vi "ni_home.vi"(8 "error in":errorcluster) -> (0 "error out":errorcluster)   [LabVIEW 2014]
uses:
  <vilib>/Motion/FlexMotion/CustomControls/CustomControls.llb/Axis # (8 axes).flx
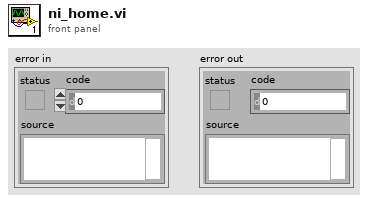
[diagram p1: front panel]
types:
  T1 = typedef "Board Id" = u8
  T2 = enum16{"Home", "Index", "Center", "Forward Limit", "Reverse Limit", "Run Sequence"}
  T3 = typedef "Axis # (8 axes).flx" = cluster{"1":bool, "2":bool, "3":bool, "4":bool, "5":bool, "6":bool, "7":bool, "8":bool}
  T4 = typedef "AxisOrVectorSpaceControl To Control.flx" = u16
  T5 = typedef "Bd Id Out" = u8
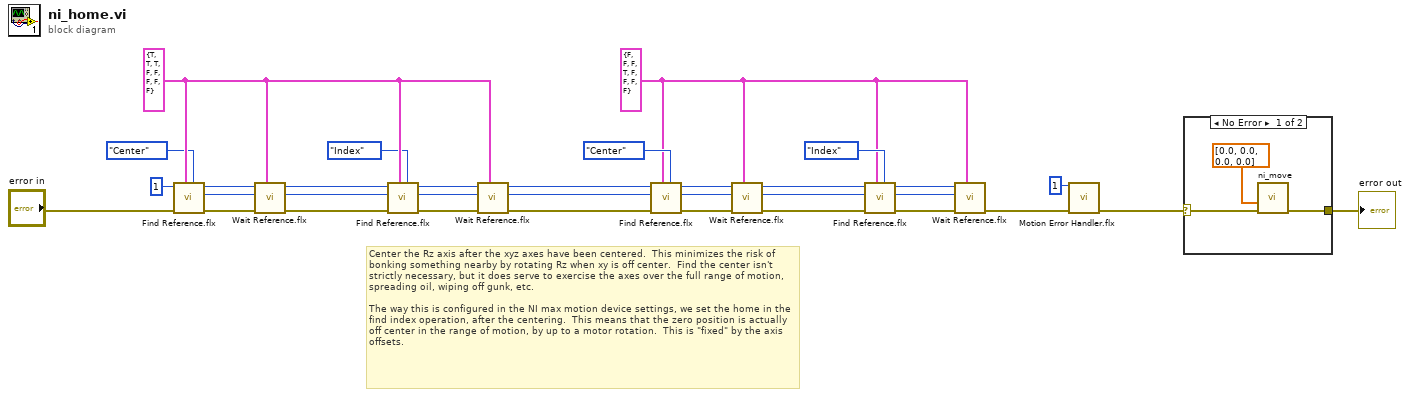
[diagram p0: block diagram]
diagram:
  w18 = T3 {"1"=FALSE, "2"=FALSE, "3"=FALSE, "4"=TRUE, "5"=FALSE, "6"=FALSE, "7"=FALSE, "8"=FALSE} ("Axis/VS Map (Disabled)")
  w17 = T3 {"1"=TRUE, "2"=TRUE, "3"=TRUE, "4"=FALSE, "5"=FALSE, "6"=FALSE, "7"=FALSE, "8"=FALSE} ("Axis/VS Map (Disabled)")
  # "Center the Rz axis after the xyz axes have been centered.  This minimizes the risk of bonking something nearby by rotating Rz when xy is off center.  Find the center isn't strictly necessary, but it does serve to exercise the axes over the full range of motion, spreading oil, wiping off gunk, etc.  \n\nThe way this is configured in the NI max motion device settings, we set the home in the find index operation, after the centering.  This means that the zero position is actually off center in the range of motion, by up to a motor rotation.  This is \"fixed\" by the axis offsets."
  n1 = call <vilib>:"Find Reference.flx"("Search Type"=T2."Center", "Axis/VS Map (Disabled)"=w17, "error in (no error)"="error in", "Board ID"=T1 1) -> ("error out"=w5:errorcluster, "Axis or Vector Space Output"=w8:T4, "Bd ID Out"=w7:T5)  [unwired: 5 in]
  n2 = call <vilib>:"Wait Reference.flx"("Axis/VS Map (Disabled)"=w17, "error in (no error)"=w5, "Axis or Vector Space"=w8, "Board ID"=w7) -> ("error out"=w11:errorcluster, "Axis or Vector Space Output"=w16:T4, "Bd ID Out"=w15:T5)  [unwired: 4 in, 1 out]
  n3 = call <vilib>:"Find Reference.flx"("Search Type"=T2."Index", "Axis/VS Map (Disabled)"=w17, "error in (no error)"=w11, "Axis or Vector Space"=w16, "Board ID"=w15) -> ("error out"=w12:errorcluster, "Axis or Vector Space Output"=w14:T4, "Bd ID Out"=w13:T5)  [unwired: 4 in]
  n4 = call <vilib>:"Wait Reference.flx"("Axis/VS Map (Disabled)"=w17, "error in (no error)"=w12, "Axis or Vector Space"=w14, "Board ID"=w13) -> ("error out"=w32:errorcluster, "Axis or Vector Space Output"=w31:T4, "Bd ID Out"=w30:T5)  [unwired: 4 in, 1 out]
  n5 = call <vilib>:"Find Reference.flx"("Search Type"=T2."Center", "Axis/VS Map (Disabled)"=w18, "error in (no error)"=w32, "Axis or Vector Space"=w31, "Board ID"=w30) -> ("error out"=w29:errorcluster, "Axis or Vector Space Output"=w27:T4, "Bd ID Out"=w28:T5)  [unwired: 4 in]
  n6 = call <vilib>:"Wait Reference.flx"("Axis/VS Map (Disabled)"=w18, "error in (no error)"=w29, "Axis or Vector Space"=w27, "Board ID"=w28) -> ("error out"=w24:errorcluster, "Axis or Vector Space Output"=w19:T4, "Bd ID Out"=w20:T5)  [unwired: 4 in, 1 out]
  n7 = call <vilib>:"Find Reference.flx"("Search Type"=T2."Index", "Axis/VS Map (Disabled)"=w18, "error in (no error)"=w24, "Axis or Vector Space"=w19, "Board ID"=w20) -> ("error out"=w23:errorcluster, "Axis or Vector Space Output"=w21:T4, "Bd ID Out"=w22:T5)  [unwired: 4 in]
  n8 = call <vilib>:"Wait Reference.flx"("Axis/VS Map (Disabled)"=w18, "error in (no error)"=w23, "Axis or Vector Space"=w21, "Board ID"=w22) -> ("error out"=w3:errorcluster)  [unwired: 4 in, 3 out]
  n9 = call <vilib>:"Motion Error Handler.flx"("Board ID"=T1 1, "error in (no error)"=w3) -> ("error out"=w2:errorcluster)  [unwired: 9 in, 4 out]
  n10 = case shown="No Error" w2 {
    selector: w2 -> [w35 w37]
    tunnel: [w34 w37] -> w1
    frame No Error {
      n11 = call "ni_move.vi"("error in"=w35, "Axis positions"=dbl[] [0.0, 0.0, 0.0, 0.0]) -> ("error out"=w34:errorcluster)  [unwired: 9 in]
    }
    frame Error {
    }
  }
  "error out" <- w1
